vi "Generate Parameter Multifit.vi"(9 "FWHM Bound Parameters (%)":dbl, 10 "EnOffsetFit":bool, 11 "All Parameter Fit":dbl[][](array[numeric])) -> (1 "Initial Conditions":dbl[](array[numeric]), 2 "Rearranged Parameter Fit":dbl[][](array[numeric]), 3 "Parameter Offset":dbl, 4 "Max Bound Condition":dbl[](array[numeric]), 6 "Min Bound Condition":dbl[](array[numeric]))   [LabVIEW 2023]
uses:
  a7cf3ec9-e608-4443-b365-49f118129d8c.vi
  <vilib>/Utility/Data Type/Get Array Information.vi
  <vilib>/Utility/Data Type/Get Type Information.vi
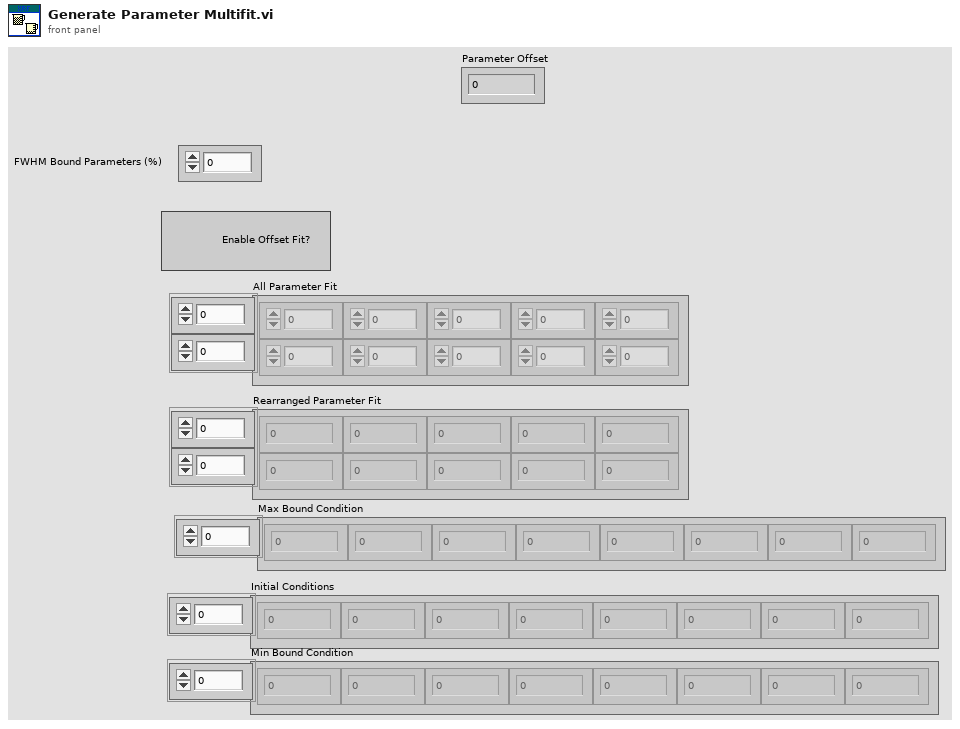
[diagram p1: front panel]
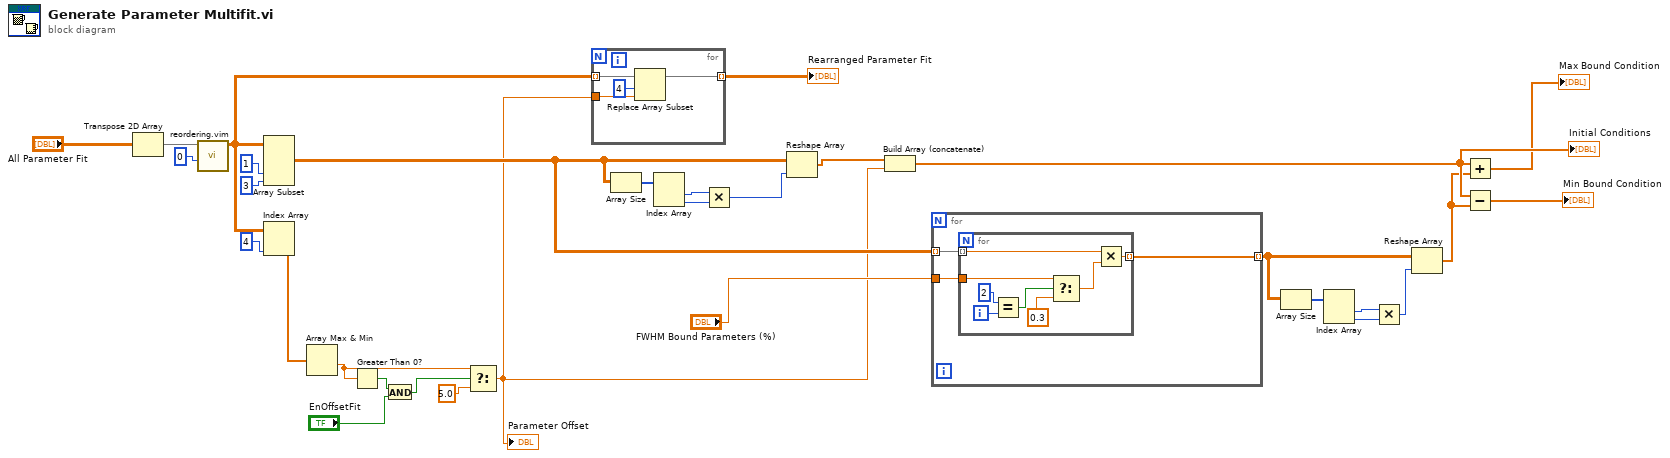
[diagram p0: block diagram]
diagram:
  n1 = Transpose 2D Array(2D array="All Parameter Fit") -> (transposed array=w31:dbl[][])
  n2 = call "reordering.vim"("Row to Reorder"=0, "Data In"=w31) -> ("Data Out"=w3:dbl[][])  [unwired: 8 in, 1 out]
  n3 = Array Subset(array=w3, index (col)=1 ("index"), length (col)=3 ("length")) -> (w13:dbl[][])  [unwired: 2 in]
  n4 = Index Array(array=w3, index (col)=4 ("disabled index (col)")) -> (element=w14:dbl[])  [unwired: 1 in]
  n5 = Array Max & Min(array=w14) -> (min value=w24:dbl)  [unwired: 3 out]
  n6 = Greater Than 0?(x=w24) -> (x > 0?=w6:bool)
  n7 = And(x=w6, y="EnOffsetFit") -> (x .and. y?=w5:bool)
  n8 = Select(t=w24, s=w5, f=5.0) -> (s? t:f=w1:dbl)
  "Parameter Offset" <- w1
  n9 = for {
    tunnel: w3 -> [w35] mode=indexing
    tunnel: w1 -> [w34]
    tunnel: [w32] -> w2 mode=indexing
    n10 = Replace Array Subset(array=w35, new element=w34, index=4) -> (w32:dbl[])
  }
  "Rearranged Parameter Fit" <- w2
  n11 = Array Size(array=w13) -> (size(s)=w18:i32[])
  n12 = Index Array(array=w18) -> (element #1=w20:i32, element #2=w19:i32)  [unwired: 2 in]
  n13 = Multiply(x=w20, y=w19) -> (x*y=w21:i32)
  n14 = Reshape Array(w13, w21) -> (w22:dbl[])
  n15 = Build Array (concatenate)(w22, w1) -> (w23:dbl[])
  "Initial Conditions" <- w23
  n16 = for {
    tunnel: "FWHM Bound Parameters (%)" -> [w38]
    tunnel: w13 -> [w37] mode=indexing
    tunnel: [w36] -> w7 mode=indexing
    n17 = for {
      tunnel: w38 -> [w44]
      tunnel: w37 -> [w42] mode=indexing
      tunnel: [w41] -> w36 mode=indexing
      i -> [w40]
      n18 = Equal?(x=2, y=w40) -> (x = y?=w45:bool)
      n19 = Select(t=w44, s=w45, f=0.3) -> (s? t:f=w43:dbl)
      n20 = Multiply(x=w42, y=w43) -> (x*y=w41:dbl)
    }
  }
  n21 = Array Size(array=w7) -> (size(s)=w12:i32[])
  n22 = Index Array(array=w12) -> (element #1=w10:i32, element #2=w11:i32)  [unwired: 2 in]
  n23 = Multiply(x=w10, y=w11) -> (x*y=w9:i32)
  n24 = Reshape Array(w7, w9) -> (w8:dbl[])
  n25 = Add(x=w23, y=w8) -> (x+y=→"Max Bound Condition":dbl[])
  n26 = Subtract(x=w23, y=w8) -> (x-y=→"Min Bound Condition":dbl[])
